vi "Setup 3D Picture Display.vi"(10 "Color":T1={"Red"=1.0, "Green"=0.0, "Blue"=0.0, "Alpha"=1.0}, 11 "Name":string) -> (1 "SceneObject out":refnum<vi>, 3 "Scene:New Object":refnum<vi>)   [LabVIEW 2014]
uses:
  <vilib>/picture/3D Picture Control/Object/Create Object (name).vi
  <vilib>/picture/3D Picture Control/NI_3D Picture Control.lvlib
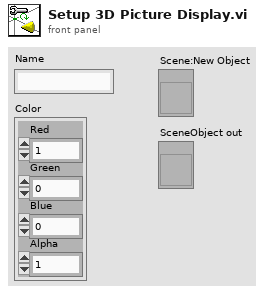
[diagram p1: front panel]
types:
  T1 = cluster{"Red":sgl, "Green":sgl, "Blue":sgl, "Alpha":sgl}
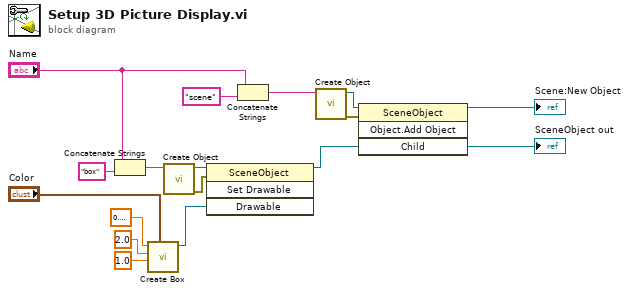
[diagram p0: block diagram]
diagram:
  n1 = Concatenate Strings("Name", "box" ("string")) -> (w4:string)
  n2 = call <vilib>:"Create Box.vi"("Color"="Color", "Length Z"=sgl 1.0, "Length Y"=sgl 2.0, "Length X"=sgl 0.2) -> ("New Box Refnum"=w12:refnum<vi>)  [unwired: 6 in, 1 out]
  n3 = call-poly <vilib>:"Create Object.vi"("Name"=w4) -> ("error out"=w11:errorcluster, "Scene:New Object"=w10:refnum<vi>)  [unwired: 9 in]
  n4 = invoke class="SceneObject" method="Set Drawable"(reference=w10, error in=w11, "Drawable"=w12) -> (reference out=w15:refnum<vi>)  [unwired: 1 in, 3 out]
  n5 = Concatenate Strings("Name", "scene" ("string")) -> (w5:string)
  n6 = call-poly <vilib>:"Create Object.vi"("Name"=w5) -> ("error out"=w14:errorcluster, "Scene:New Object"=w13:refnum<vi>)  [unwired: 9 in]
  n7 = invoke class="SceneObject" method="Object.Add Object"(reference=w13, error in=w14, "Child"=w15) -> (reference out=→"Scene:New Object":refnum<vi>, "Child"=→"SceneObject out":refnum<vi>)  [unwired: 1 in, 2 out]
